vi "SerialVoltage.vi"() -> ()   [LabVIEW 2015]
doc: "本范例根据用户指示，对串口执行读写操作。范例运行时可按下“写入”或“读取”按钮，以及修改“读数”。\n\n设置的串口参数必须匹配连接仪器或设备的参数。本范例中，“读数”参数可指定串口读取的字节数。如端口字节超过指定的字节数，超出部分将不会被读取。如端口字节数少于指定的字节数，将返回超时错误。\n\n本范例可扩展流控制选项以包括XON和XOFF，从而允许用户选择控制字符。同时，用户可启用或禁用中止符。部分设备需要通过终止符确定命令字符串的结束位置。部分设备将发送终止符以说明待读取数据的末端。本范例演示了缓冲区中检测到终止符时，结束“读取”操作或添加终止符至“写入”数据末端的方法。"
uses:
  C:/Program Files (x86)/National Instruments/LabVIEW 2015/examples/Instrument IO/Serial/support/Serial - Settings.ctl
  <vilib>/Instr/_visa.llb/VISA Configure Serial Port (Instr).vi
panel:
  out "电压":dbl(knob) scale=0.0..5.0
  in  "停止":bool
  in  "VISA资源名称":refnum<visa-resource-name>="COM1"
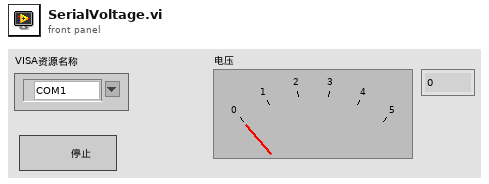
[diagram p1: front panel]
types:
  T1 = typedef "Serial - Settings.ctl" = cluster{"波特率":u32, "数据比特":u16, "奇偶":enum16{"None", "Odd", "Even", "Mark", "Space"}, "停止位":u16, "流控制":u16}
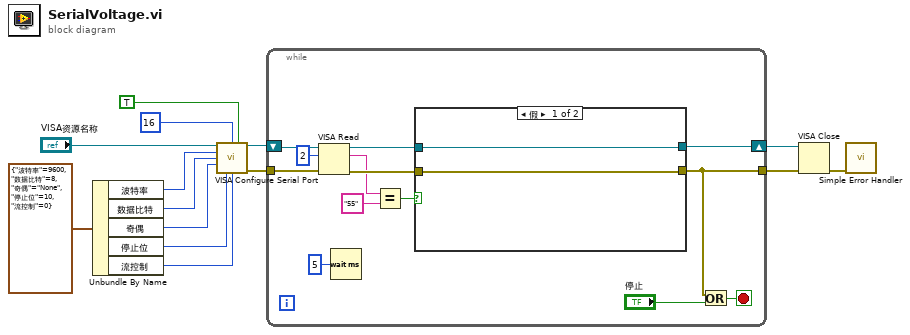
[diagram p0: block diagram]
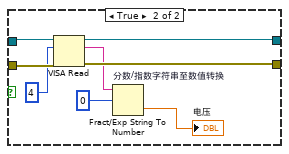
[diagram p2: hidden frame]
diagram:
  n1 = Unbundle By Name(T1 {"波特率"=9600, "数据比特"=8, "奇偶"=enum."None", "停止位"=10, "流控制"=0} ("串口设置")) -> ("波特率"=w11:u32, "数据比特"=w12:u16, "奇偶"=w13:enum16{"None", "Odd", "Even", "Mark", "Space"}, "停止位"=w14:u16, "流控制"=w5:u16)
  n2 = call-poly "VISA Configure Serial Port"("VISA resource name"="VISA资源名称", "termination char\n(0xA = '\\n' = LF)"=u8 16 ("终止符"), "Enable Termination\nChar (T)"=TRUE ("终止符时结束读取？"), "baud rate (9600)"=w11, "data bits (8)"=w12, "parity (0:none)"=w13, "stop bits (10: 1 bit)"=w14, "flow control (0:none)"=w5) -> ("VISA resource name out"=w3:refnum<visa-resource-name>, "error out"=w4:errorcluster)  [unwired: 2 in, 4 out]
  n3 = while {
    shift-right: [w24] -> w6
    shift-left: w3 -> [w23]
    tunnel: w4 -> [w22]
    tunnel: [w15] -> w7
    stop <- w26 stop-if-true
    n4 = VISA Read(VISA resource name=w23, byte count=u32 2 ("字节总数"), error in (no error)=w22) -> (VISA resource name out=w20:refnum<visa-resource-name>, read buffer=w18:string, error out=w19:errorcluster)  [unwired: 1 out]
    n5 = Wait (ms)(milliseconds to wait=u32 5) -> ()  [unwired: 1 out]
    n6 = Equal?(x=w18, y="55") -> (x = y?=w16:bool)
    n7 = case shown="假" w16 {
      tunnel: [w29 w34] -> w24
      tunnel: [w28 w33] -> w15
      tunnel: w20 -> [w29 w37]
      tunnel: w19 -> [w28 w36]
      frame False {
      }
      frame True {
        n8 = VISA Read(VISA resource name=w37, byte count=u32 4 ("字节总数"), error in (no error)=w36) -> (VISA resource name out=w34:refnum<visa-resource-name>, read buffer=w32:string, error out=w33:errorcluster)  [unwired: 1 out]
        n9 = Fract/Exp String To Number "分数/指数字符串至数值转换"(string=w32, offset=0 ("偏移量")) -> (number=→"电压":dbl)  [unwired: 2 in, 1 out]
      }
    }
    n10 = Or(x=w15, y="停止") -> (x .or. y?=w26:bool)
  }
  n11 = VISA Close(VISA resource name=w6, error in (no error)=w7) -> (error out=w8:errorcluster)
  n12 = call <vilib>:"Simple Error Handler.vi"("error in (no error)"=w8) -> ()  [unwired: 1 in, 8 out]
